vi "report file error.vi"(8 "failure in":T1 {"code" format="%.0x"}, 10 "file path":path, 11 "error in":errorcluster) -> (0 "failure":T1 {"code" format="%.0x"})   [LabVIEW 2013, in "file errors.lvlib"]
uses:
  file errors.lvlib
  failure.ctl
  const exceptioncausename.vi
  const severityname.vi
  Variant Repository/Write Variant Repository/Write Exception Property.xnode
  failure.lvlib
  <vilib>/Utility/VariantDataType/GetTypeInfo.vi
  <vilib>/Utility/VariantDataType/VariantType.lvlib
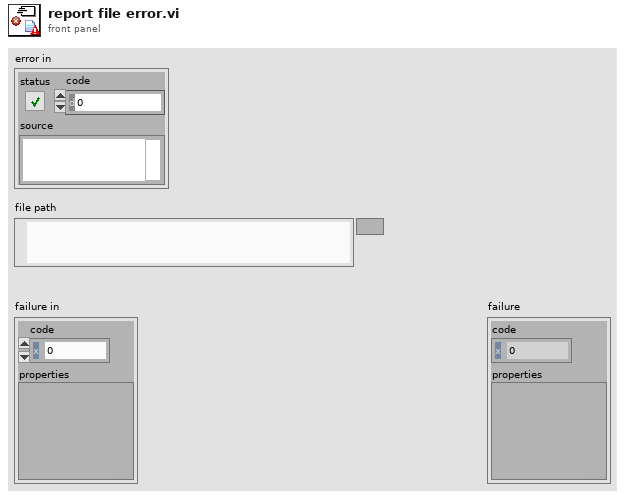
[diagram p1: front panel]
types:
  T1 = typedef "failure.lvlib/failure.ctl" = cluster{"code":i32, "properties":variant}
  T2 = typedef "failure.lvlib/severity.ctl" = enum8{"unspecified", "informational", "operation failed", "data corruption", "system corruption", "critical unknown state"}
  T3 = typedef "file errors.lvlib/file error.ctl" = enum16{"invalid path or reference", "end of file", "file already opened", "generic file error", "file not found", "permissions invalid", "disk full", "duplicate path", "too many open file handles", "useless generic error"}
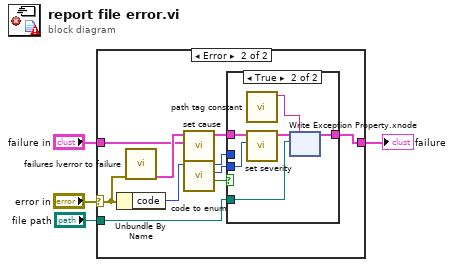
[diagram p0: block diagram]
diagram:
  n1 = case shown="Error" "error in" {
    selector: "error in" -> [_ w9]
    tunnel: "failure in" -> [w5 w7]
    tunnel: [w5 w15] -> w3
    tunnel: "file path" -> [_ w14]
    frame No Error {
    }
    frame Error {
      n2 = Unbundle By Name(w9) -> ("code"=w13:i32)
      n3 = call "failures lverror to failure.vi"("error in"=w9) -> ("failure"=w8:T1)  [unwired: 10 in]
      n4 = call "set cause.vi"("cause"=w7, "failure in"=w8) -> ("failure out"=w6:T1)  [unwired: 9 in]
      n5 = call "code to enum.vi"("code"=w13) -> ("valid?"=w12:bool, "severity"=w11:T2, "file error"=w10:T3)  [unwired: 8 in]
      n6 = case shown="True" w12 {
        tunnel: w6 -> [w16 w19]
        tunnel: [w16 w18] -> w15
        tunnel: w14 -> [_ w17]
        tunnel: w11 -> [_ w21]
        tunnel: w10 -> [_ _]
        frame False {
        }
        frame True {
          n7 = call "path tag constant.vi"() -> ("Tag"=w22:string)  [unwired: 11 in]
          n8 = call "set severity.vi"("severity"=w21, "failure in"=w19) -> ("failure out"=w20:T1)  [unwired: 9 in]
          n9 = xnode "Write Exception Property.xnode"("error reporter in"=w20, "Tag"=w22, "Value"=w17) -> ("error reporter out"=w18:T1)  [unwired: 1 out]
        }
      }
    }
  }
  "failure" <- w3
